vi "R567X_CAN高级功能.vi"() -> ()   [LabVIEW 2020]
panel:
  out "B'":i16
  out "B":i16
  out "A":i16
  out "A'":i16
  out "OK":bool caption="启动标定成功"
  out "完成":bool caption="启动标定成功"
  out "标定成功":bool caption="启动标定成功"
  out "当前扭矩":dbl
  out "扭矩已标定":bool
  out "当前角度":dbl
  out "角度已标定":bool
  out "Out_Time":bool
  in  "error in":errorcluster
  in  "Function":T1(ring)
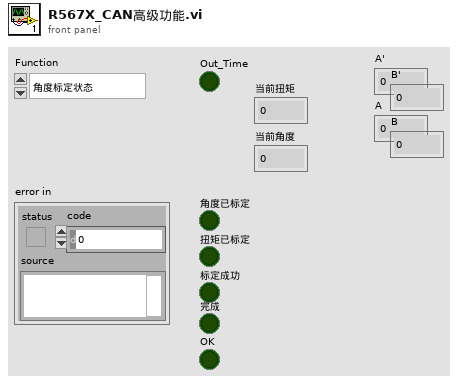
[diagram p1: front panel]
types:
  T1 = enum16{"角度标定状态", "角度标定", "角度标定清除", "扭矩标定状态", "扭矩标定", "扭矩标定清除", "内部软件版本号", "客户软件版本号"}
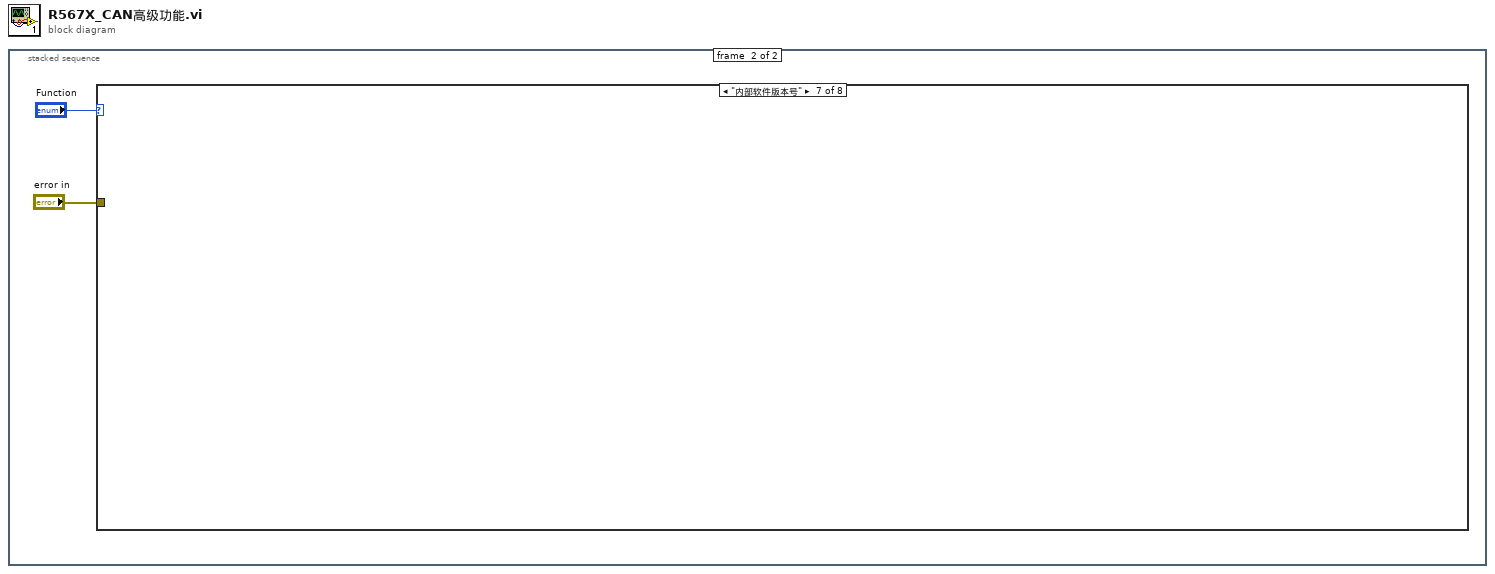
[diagram p0: block diagram]
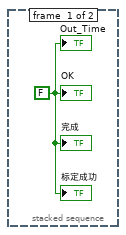
[diagram p2: hidden frame]
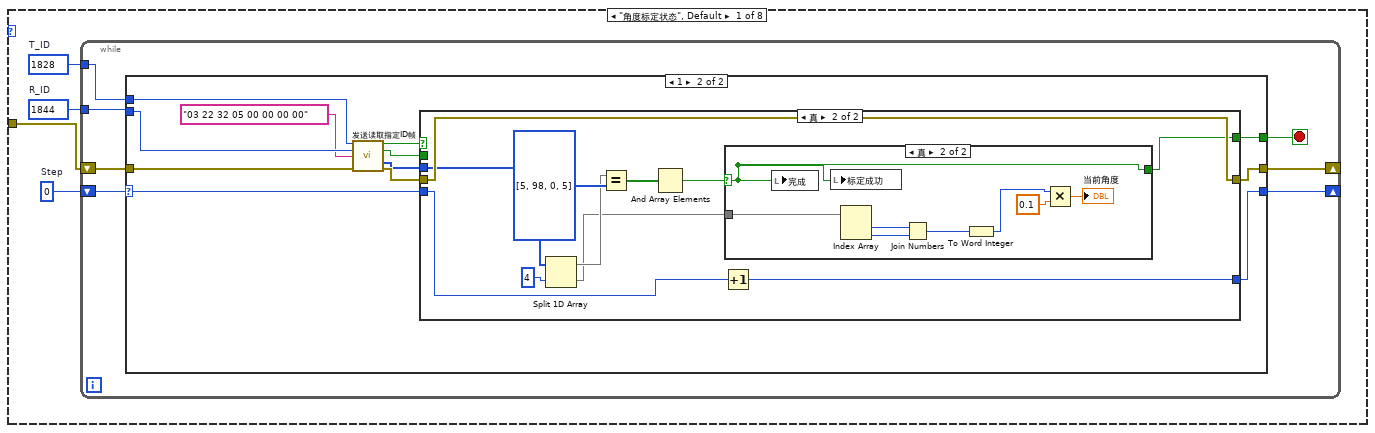
[diagram p3: hidden frame]
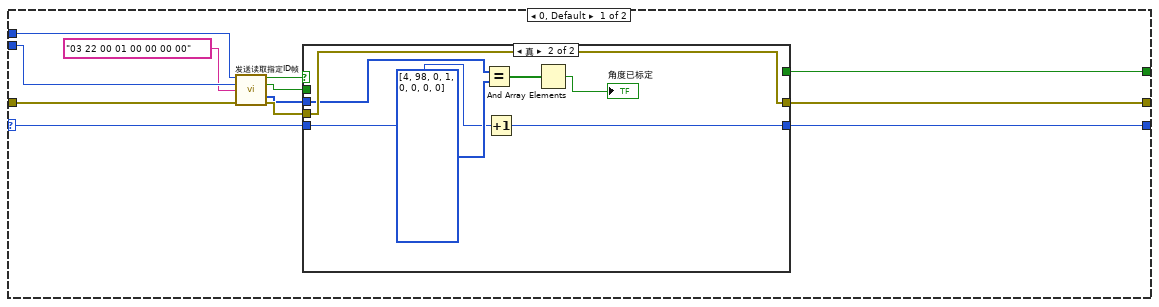
[diagram p4: hidden frame]
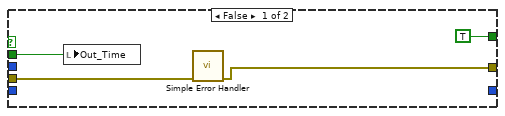
[diagram p5: hidden frame]
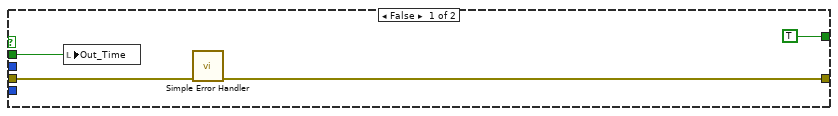
[diagram p6: hidden frame]
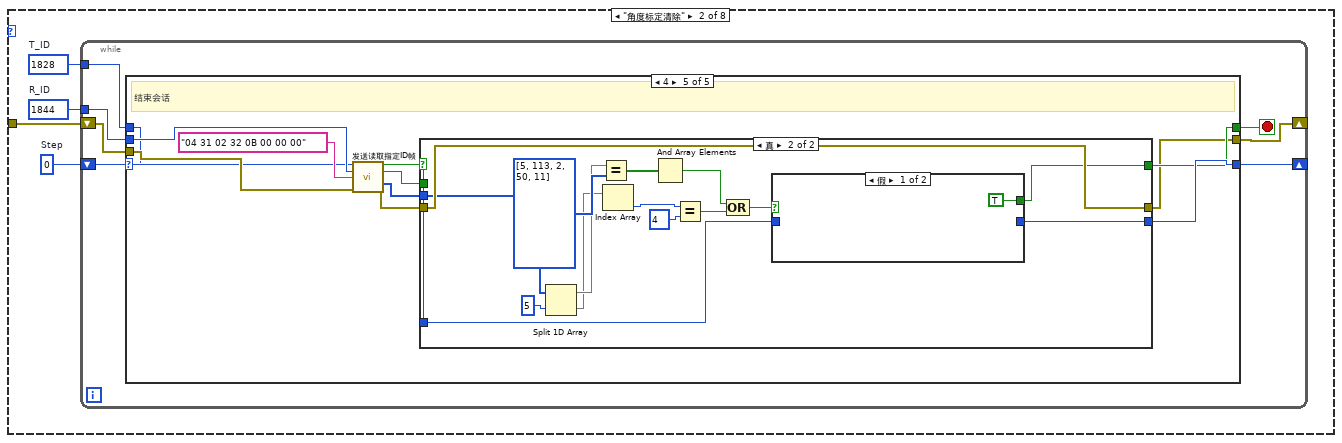
[diagram p8: hidden frame]
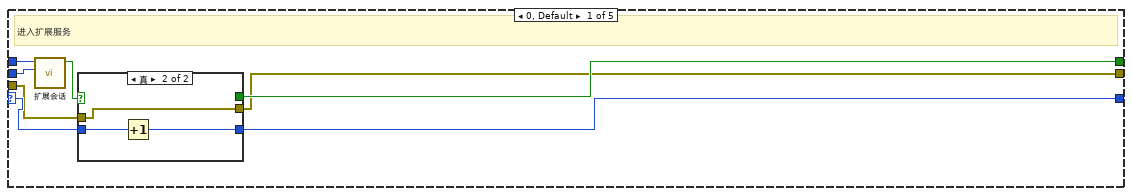
[diagram p9: hidden frame]
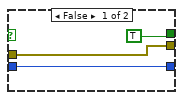
[diagram p10: hidden frame]
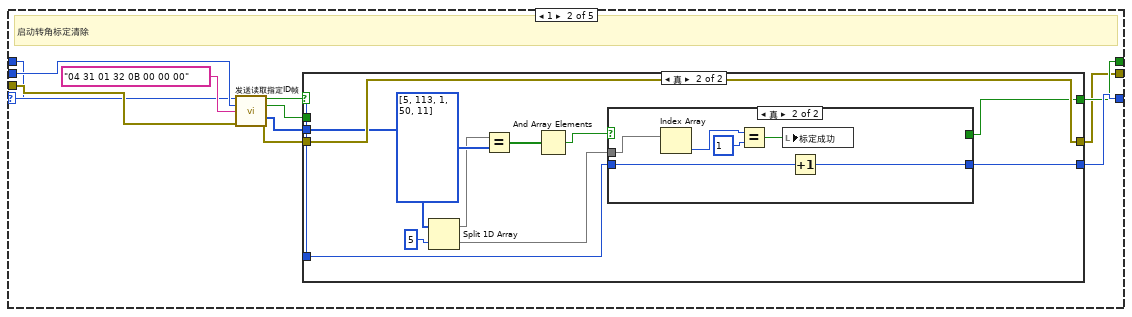
[diagram p11: hidden frame]
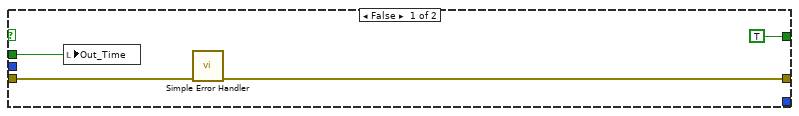
[diagram p12: hidden frame]
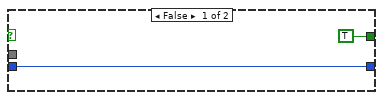
[diagram p13: hidden frame]
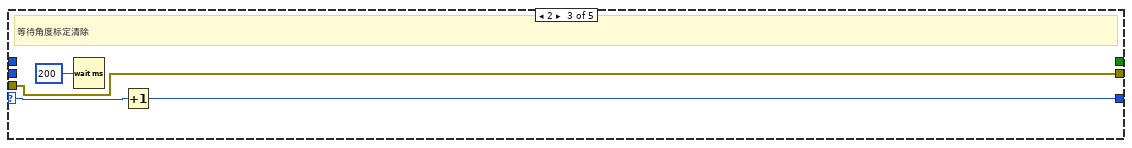
[diagram p14: hidden frame]
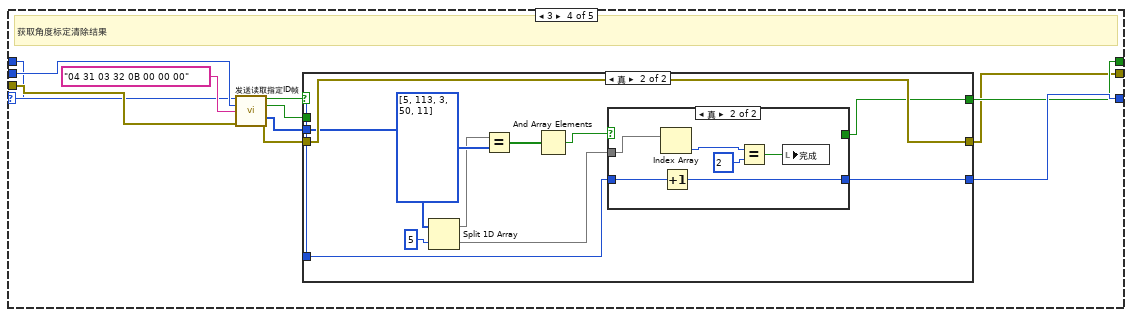
[diagram p15: hidden frame]
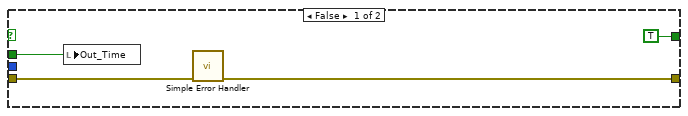
[diagram p16: hidden frame]
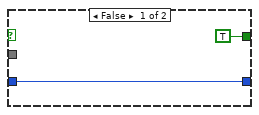
[diagram p17: hidden frame]
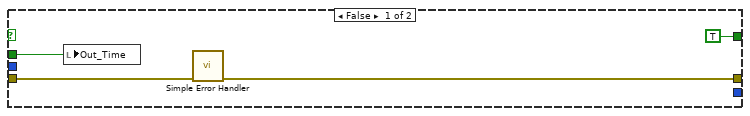
[diagram p18: hidden frame]
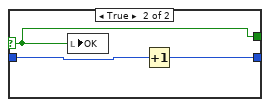
[diagram p19: hidden frame]
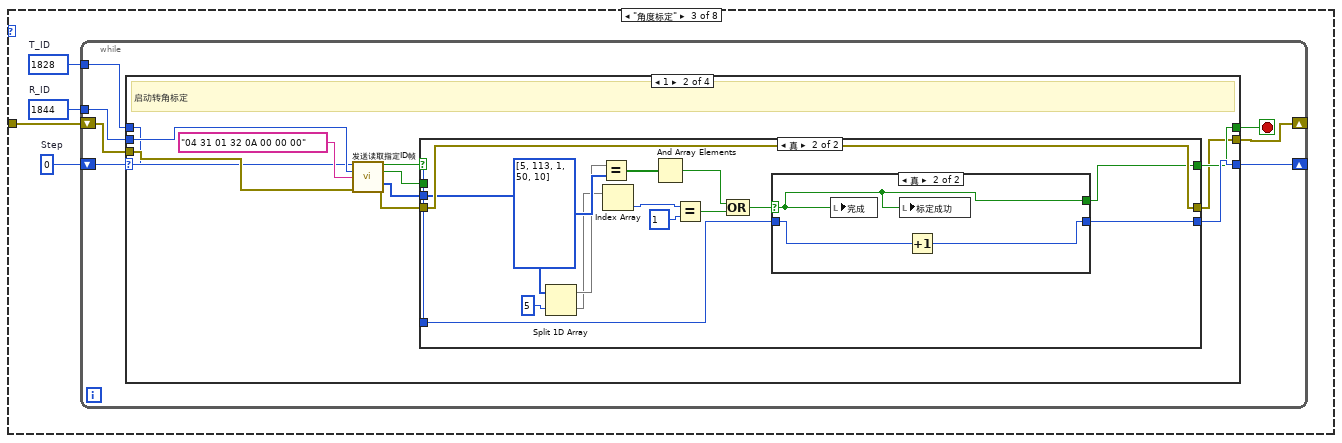
[diagram p20: hidden frame]
diagram:
  n1 = stacked-sequence {
    frame #0 {
      w1 = FALSE ("Out_Time")
      "Out_Time" <- w1
      "标定成功" <- w1
      "完成" <- w1
      "OK" <- w1
    }
    frame #1 {
      n2 = case shown="\"内部软件版本号\"" "Function" {
        tunnel: "error in" -> [w7 w73 w207 w311 w377 w605 _ _]
        frame "角度标定状态", Default {
          w4 = u32 1828  # T_ID
          w5 = u32 1844  # R_ID
          w6 = 0  # Step
          n3 = while {
            tunnel: w4 -> [w14]
            tunnel: w5 -> [w12]
            shift-right: [w8] -> _
            shift-left: w6 -> [w11]
            shift-right: [w9] -> _
            shift-left: w7 -> [w13]
            stop <- w10 stop-if-true
            n4 = case shown="1" w11 {
              selector: w11 -> [w16 w39]
              tunnel: w14 -> [w26 w49]
              tunnel: w13 -> [w25 w48]
              tunnel: w12 -> [w24 w47]
              tunnel: [w20 w43] -> w10
              tunnel: [w18 w41] -> w9
              tunnel: [w15 w38] -> w8
              frame 0, Default {
                n5 = call "发送读取指定ID帧.vi"("T_ID"=w26, "R_ID"=w24, "CAN_Frame"="03 22 00 01 00 00 00 00", "error in (no error)"=w25) -> ("OK"=w22:bool, "Out_Time"=w21:bool, "Recive"=w17:u8[], "error out"=w19:errorcluster)  [unwired: 7 in, 1 out]
                n6 = case shown="真" w22 {
                  tunnel: w21 -> [w30 _]
                  tunnel: [TRUE _] -> w20
                  tunnel: w19 -> [w28 w37]
                  tunnel: [w27 w37] -> w18
                  tunnel: w17 -> [_ w36]
                  tunnel: w16 -> [_ w32]
                  tunnel: [_ w31] -> w15
                  frame False {
                    n7 = local write "Out_Time"(w30) -> ()
                    n8 = call <vilib>:"Simple Error Handler.vi"("error in (no error)"=w28) -> ("error out"=w27:errorcluster)  [unwired: 4 in, 4 out]
                  }
                  frame True {
                    n9 = Equal?(x=w36, y=u8[] [4, 98, 0, 1, 0, 0, 0, 0]) -> (x = y?=w34:bool[])
                    n10 = Increment(x=w32) -> (x+1=w31:i32)
                    n11 = And Array Elements(Boolean array=w34) -> (logical AND=→"角度已标定":bool)
                  }
                }
              }
              frame 1 {
                n12 = call "发送读取指定ID帧.vi"("T_ID"=w49, "R_ID"=w47, "CAN_Frame"="03 22 32 05 00 00 00 00", "error in (no error)"=w48) -> ("OK"=w45:bool, "Out_Time"=w44:bool, "Recive"=w40:u8[], "error out"=w42:errorcluster)  [unwired: 7 in, 1 out]
                n13 = case shown="真" w45 {
                  tunnel: w44 -> [w53 _]
                  tunnel: [TRUE w54] -> w43
                  tunnel: w42 -> [w51 w64]
                  tunnel: [w50 w64] -> w41
                  tunnel: w40 -> [_ w59]
                  tunnel: w39 -> [_ w61]
                  tunnel: [_ w60] -> w38
                  frame False {
                    n14 = local write "Out_Time"(w53) -> ()
                    n15 = call <vilib>:"Simple Error Handler.vi"("error in (no error)"=w51) -> ("error out"=w50:errorcluster)  [unwired: 4 in, 4 out]
                  }
                  frame True {
                    n16 = Split 1D Array(array=w59, index=4 ("索引")) -> (first subarray=w57:u8[], second subarray=w56:u8[])
                    n17 = Equal?(x=w57, y=u8[] [5, 98, 0, 5]) -> (x = y?=w62:bool[])
                    n18 = And Array Elements(Boolean array=w62) -> (logical AND=w55:bool)
                    n19 = Increment(x=w61) -> (x+1=w60:i32)
                    n20 = case shown="真" w55 {
                      selector: w55 -> [_ w65]
                      tunnel: w56 -> [_ w72]
                      tunnel: [_ w65] -> w54
                      frame False {
                      }
                      frame True {
                        n21 = local write "完成"(w65) -> ()
                        n22 = local write "标定成功"(w65) -> ()
                        n23 = Index Array(array=w72) -> (element #1=w70:u8, element #2=w71:u8)  [unwired: 2 in]
                        n24 = Join Numbers(hi=w70, lo=w71) -> ((hi.lo)=w67:u16)
                        n25 = To Word Integer(number=w67) -> (16bit integer=w66:i16)
                        n26 = Multiply(x=w66, y=0.1) -> (x*y=→"当前角度":dbl)
                      }
                    }
                  }
                }
              }
            }
          }
        }
        frame "角度标定清除" {
          w76 = u32 1828  # T_ID
          w75 = u32 1844  # R_ID
          w74 = 0  # Step
          n27 = while {
            tunnel: w76 -> [w83]
            tunnel: w75 -> [w81]
            shift-right: [w77] -> _
            shift-left: w74 -> [w80]
            shift-right: [w78] -> _
            shift-left: w73 -> [w82]
            stop <- w79 stop-if-true
            n28 = case shown="4" w80 {
              selector: w80 -> [w88 w102 w135 w141 w176]
              tunnel: w83 -> [w91 w101 _ w140 w175]
              tunnel: w82 -> [w85 w103 w133 w142 w177]
              tunnel: w81 -> [w90 w104 _ w143 w178]
              tunnel: [w86 w99 _ w138 w173] -> w79
              tunnel: [w84 w98 w133 w137 w172] -> w78
              tunnel: [w87 w100 w134 w139 w174] -> w77
              frame 0, Default {
                # "进入扩展服务"
                n29 = call "扩展会话.vi"("R_ID"=w90, "T_ID"=w91) -> ("OK"=w89:bool)  [unwired: 8 in, 1 out]
                n30 = case shown="真" w89 {
                  tunnel: w88 -> [w94 w97]
                  tunnel: [w94 w96] -> w87
                  tunnel: [TRUE _] -> w86
                  tunnel: [w92 w95] -> w84
                  tunnel: w85 -> [w92 w95]
                  frame False {
                  }
                  frame True {
                    n31 = Increment(x=w97) -> (x+1=w96:i32)
                  }
                }
              }
              frame 1 {
                # "启动转角标定清除"
                n32 = call "发送读取指定ID帧.vi"("T_ID"=w101, "R_ID"=w104, "CAN_Frame"="04 31 01 32 0B 00 00 00", "error in (no error)"=w103) -> ("OK"=w109:bool, "Out_Time"=w108:bool, "Recive"=w106:u8[], "error out"=w107:errorcluster)  [unwired: 7 in, 1 out]
                n33 = case shown="真" w109 {
                  tunnel: w108 -> [w113 _]
                  tunnel: [TRUE w114] -> w99
                  tunnel: w107 -> [w111 w124]
                  tunnel: [w110 w124] -> w98
                  tunnel: w106 -> [_ w121]
                  tunnel: w102 -> [_ w116]
                  tunnel: [_ w115] -> w100
                  frame False {
                    n34 = local write "Out_Time"(w113) -> ()
                    n35 = call <vilib>:"Simple Error Handler.vi"("error in (no error)"=w111) -> ("error out"=w110:errorcluster)  [unwired: 4 in, 4 out]
                  }
                  frame True {
                    n36 = Split 1D Array(array=w121, index=5 ("索引")) -> (first subarray=w119:u8[], second subarray=w118:u8[])
                    n37 = Equal?(x=w119, y=u8[] [5, 113, 1, 50, 11]) -> (x = y?=w122:bool[])
                    n38 = And Array Elements(Boolean array=w122) -> (logical AND=w117:bool)
                    n39 = case shown="真" w117 {
                      tunnel: w118 -> [_ w132]
                      tunnel: w116 -> [w126 w129]
                      tunnel: [w126 w128] -> w115
                      tunnel: [TRUE _] -> w114
                      frame False {
                      }
                      frame True {
                        n40 = Index Array(array=w132) -> (element=w131:u8)  [unwired: 1 in]
                        n41 = Equal?(x=w131, y=u8 1) -> (x = y?=w127:bool)
                        n42 = local write "标定成功"(w127) -> ()
                        n43 = Increment(x=w129) -> (x+1=w128:i32)
                      }
                    }
                  }
                }
              }
              frame 2 {
                # "等待角度标定清除"
                n44 = Wait (ms)(milliseconds to wait=u32 200 ("等待时间（毫秒）")) -> ()  [unwired: 1 out]
                n45 = Increment(x=w135) -> (x+1=w134:i32)
              }
              frame 3 {
                # "获取角度标定清除结果"
                n46 = call "发送读取指定ID帧.vi"("T_ID"=w140, "R_ID"=w143, "CAN_Frame"="04 31 03 32 0B 00 00 00", "error in (no error)"=w142) -> ("OK"=w148:bool, "Out_Time"=w147:bool, "Recive"=w145:u8[], "error out"=w146:errorcluster)  [unwired: 7 in, 1 out]
                n47 = case shown="真" w148 {
                  tunnel: w147 -> [w152 _]
                  tunnel: [TRUE w153] -> w138
                  tunnel: w146 -> [w150 w163]
                  tunnel: [w149 w163] -> w137
                  tunnel: w145 -> [_ w160]
                  tunnel: w141 -> [_ w155]
                  tunnel: [_ w154] -> w139
                  frame False {
                    n48 = local write "Out_Time"(w152) -> ()
                    n49 = call <vilib>:"Simple Error Handler.vi"("error in (no error)"=w150) -> ("error out"=w149:errorcluster)  [unwired: 4 in, 4 out]
                  }
                  frame True {
                    n50 = Split 1D Array(array=w160, index=5 ("索引")) -> (first subarray=w158:u8[], second subarray=w157:u8[])
                    n51 = Equal?(x=w158, y=u8[] [5, 113, 3, 50, 11]) -> (x = y?=w161:bool[])
                    n52 = And Array Elements(Boolean array=w161) -> (logical AND=w156:bool)
                    n53 = case shown="真" w156 {
                      tunnel: w157 -> [_ w171]
                      tunnel: w155 -> [w165 w168]
                      tunnel: [w165 w167] -> w154
                      tunnel: [TRUE _] -> w153
                      frame False {
                      }
                      frame True {
                        n54 = Index Array(array=w171) -> (element=w170:u8)  [unwired: 1 in]
                        n55 = Increment(x=w168) -> (x+1=w167:i32)
                        n56 = Equal?(x=w170, y=u8 2) -> (x = y?=w166:bool)
                        n57 = local write "完成"(w166) -> ()
                      }
                    }
                  }
                }
              }
              frame 4 {
                # "结束会话"
                n58 = call "发送读取指定ID帧.vi"("T_ID"=w175, "R_ID"=w178, "CAN_Frame"="04 31 02 32 0B 00 00 00", "error in (no error)"=w177) -> ("OK"=w183:bool, "Out_Time"=w182:bool, "Recive"=w180:u8[], "error out"=w181:errorcluster)  [unwired: 7 in, 1 out]
                n59 = case shown="真" w183 {
                  tunnel: w182 -> [w187 _]
                  tunnel: [TRUE w195] -> w173
                  tunnel: w181 -> [w185 w202]
                  tunnel: [w184 w202] -> w172
                  tunnel: w180 -> [_ w199]
                  tunnel: w176 -> [_ w191]
                  tunnel: [_ w190] -> w174
                  frame False {
                    n60 = local write "Out_Time"(w187) -> ()
                    n61 = call <vilib>:"Simple Error Handler.vi"("error in (no error)"=w185) -> ("error out"=w184:errorcluster)  [unwired: 4 in, 4 out]
                  }
                  frame True {
                    n62 = Split 1D Array(array=w199, index=5 ("索引")) -> (first subarray=w197:u8[], second subarray=w192:u8[])
                    n63 = Equal?(x=w197, y=u8[] [5, 113, 2, 50, 11]) -> (x = y?=w200:bool[])
                    n64 = Index Array(array=w192) -> (element=w194:u8)  [unwired: 1 in]
                    n65 = And Array Elements(Boolean array=w200) -> (logical AND=w196:bool)
                    n66 = Equal?(x=w194, y=u8 4) -> (x = y?=w188:bool)
                    n67 = Compound Arithmetic op=OR ("复合运算")(w196, w188) -> (w189:bool)
                    n68 = case shown="假" w189 {
                      selector: w189 -> [_ w206]
                      tunnel: [TRUE w206] -> w195
                      tunnel: w191 -> [_ w205]
                      tunnel: [_ w204] -> w190
                      frame False {
                      }
                      frame True {
                        n69 = local write "OK"(w206) -> ()
                        n70 = Increment(x=w205) -> (x+1=w204:i32)
                      }
                    }
                  }
                }
              }
            }
          }
        }
        frame "角度标定" {
          w210 = u32 1828  # T_ID
          w209 = u32 1844  # R_ID
          w208 = 0  # Step
          n71 = while {
            tunnel: w210 -> [w217]
            tunnel: w209 -> [w215]
            shift-right: [w211] -> _
            shift-left: w208 -> [w214]
            shift-right: [w212] -> _
            shift-left: w207 -> [w216]
            stop <- w213 stop-if-true
            n72 = case shown="1" w214 {
              selector: w214 -> [w222 w236 w270 w276]
              tunnel: w217 -> [w225 w235 _ w275]
              tunnel: w216 -> [w219 w237 w268 w277]
              tunnel: w215 -> [w224 w238 _ w278]
              tunnel: [w220 w233 _ w273] -> w213
              tunnel: [w218 w232 w268 w272] -> w212
              tunnel: [w221 w234 w269 w274] -> w211
              frame 0, Default {
                # "进入扩展服务"
                n73 = call "扩展会话.vi"("R_ID"=w224, "T_ID"=w225) -> ("OK"=w223:bool)  [unwired: 8 in, 1 out]
                n74 = case shown="真" w223 {
                  tunnel: w222 -> [w228 w231]
                  tunnel: [w228 w230] -> w221
                  tunnel: [TRUE _] -> w220
                  tunnel: [w226 w229] -> w218
                  tunnel: w219 -> [w226 w229]
                  frame False {
                  }
                  frame True {
                    n75 = Increment(x=w231) -> (x+1=w230:i32)
                  }
                }
              }
              frame 1 {
                # "启动转角标定"
                n76 = call "发送读取指定ID帧.vi"("T_ID"=w235, "R_ID"=w238, "CAN_Frame"="04 31 01 32 0A 00 00 00", "error in (no error)"=w237) -> ("OK"=w243:bool, "Out_Time"=w242:bool, "Recive"=w240:u8[], "error out"=w241:errorcluster)  [unwired: 7 in, 1 out]
                n77 = case shown="真" w243 {
                  tunnel: w242 -> [w247 _]
                  tunnel: [TRUE w253] -> w233
                  tunnel: w241 -> [w245 w262]
                  tunnel: [w244 w262] -> w232
                  tunnel: w240 -> [_ w259]
                  tunnel: w236 -> [_ w255]
                  tunnel: [_ w254] -> w234
                  frame False {
                    n78 = local write "Out_Time"(w247) -> ()
                    n79 = call <vilib>:"Simple Error Handler.vi"("error in (no error)"=w245) -> ("error out"=w244:errorcluster)  [unwired: 4 in, 4 out]
                  }
                  frame True {
                    n80 = Split 1D Array(array=w259, index=5 ("索引")) -> (first subarray=w257:u8[], second subarray=w250:u8[])
                    n81 = Equal?(x=w257, y=u8[] [5, 113, 1, 50, 10]) -> (x = y?=w260:bool[])
                    n82 = Index Array(array=w250) -> (element=w252:u8)  [unwired: 1 in]
                    n83 = And Array Elements(Boolean array=w260) -> (logical AND=w256:bool)
                    n84 = Equal?(x=w252, y=u8 1) -> (x = y?=w248:bool)
                    n85 = Compound Arithmetic op=OR ("复合运算")(w256, w248) -> (w249:bool)
                    n86 = case shown="真" w249 {
                      selector: w249 -> [_ w265]
                      tunnel: w255 -> [w264 w267]
                      tunnel: [w264 w266] -> w254
                      tunnel: [TRUE w265] -> w253
                      frame False {
                      }
                      frame True {
                        n87 = local write "完成"(w265) -> ()
                        n88 = local write "标定成功"(w265) -> ()
                        n89 = Increment(x=w267) -> (x+1=w266:i32)
                      }
                    }
                  }
                }
              }
              frame 2 {
                # "等待角度标定"
                n90 = Wait (ms)(milliseconds to wait=u32 200 ("等待时间（毫秒）")) -> ()  [unwired: 1 out]
                n91 = Increment(x=w270) -> (x+1=w269:i32)
              }
              frame 3 {
                # "获取角度标定结果"
                n92 = call "发送读取指定ID帧.vi"("T_ID"=w275, "R_ID"=w278, "CAN_Frame"="04 31 02 32 0A 00 00 00", "error in (no error)"=w277) -> ("OK"=w283:bool, "Out_Time"=w282:bool, "Recive"=w280:u8[], "error out"=w281:errorcluster)  [unwired: 7 in, 1 out]
                n93 = case shown="真" w283 {
                  tunnel: w282 -> [w287 _]
                  tunnel: [TRUE w288] -> w273
                  tunnel: w281 -> [w285 w298]
                  tunnel: [w284 w298] -> w272
                  tunnel: w280 -> [_ w295]
                  tunnel: w276 -> [_ w290]
                  tunnel: [_ w289] -> w274
                  frame False {
                    n94 = local write "Out_Time"(w287) -> ()
                    n95 = call <vilib>:"Simple Error Handler.vi"("error in (no error)"=w285) -> ("error out"=w284:errorcluster)  [unwired: 4 in, 4 out]
                  }
                  frame True {
                    n96 = Split 1D Array(array=w295, index=5 ("索引")) -> (first subarray=w293:u8[], second subarray=w292:u8[])
                    n97 = Equal?(x=w293, y=u8[] [5, 113, 2, 50, 10]) -> (x = y?=w296:bool[])
                    n98 = And Array Elements(Boolean array=w296) -> (logical AND=w291:bool)
                    n99 = case shown="真" w291 {
                      tunnel: w292 -> [_ w307]
                      tunnel: w290 -> [w300 w304]
                      tunnel: [w300 w303] -> w289
                      tunnel: [TRUE TRUE] -> w288
                      frame False {
                      }
                      frame True {
                        n100 = Index Array(array=w307) -> (element=w306:u8)  [unwired: 1 in]
                        n101 = Increment(x=w304) -> (x+1=w303:i32)
                        n102 = Equal?(x=w306, y=u8 4) -> (x = y?=w302:bool)
                        n103 = local write "完成"(w302) -> ()
                      }
                    }
                  }
                }
              }
            }
          }
        }
        frame "扭矩标定状态" {
          w308 = u32 1828  # T_ID
          w309 = u32 1844  # R_ID
          w310 = 0  # Step
          n104 = while {
            tunnel: w308 -> [w318]
            tunnel: w309 -> [w316]
            shift-right: [w312] -> _
            shift-left: w310 -> [w315]
            shift-right: [w313] -> _
            shift-left: w311 -> [w317]
            stop <- w314 stop-if-true
            n105 = case shown="1" w315 {
              selector: w315 -> [w320 w343]
              tunnel: w318 -> [w330 w353]
              tunnel: w317 -> [w329 w352]
              tunnel: w316 -> [w328 w351]
              tunnel: [w324 w347] -> w314
              tunnel: [w322 w345] -> w313
              tunnel: [w319 w342] -> w312
              frame 0, Default {
                n106 = call "发送读取指定ID帧.vi"("T_ID"=w330, "R_ID"=w328, "CAN_Frame"="03 22 00 05 00 00 00 00", "error in (no error)"=w329) -> ("OK"=w326:bool, "Out_Time"=w325:bool, "Recive"=w321:u8[], "error out"=w323:errorcluster)  [unwired: 7 in, 1 out]
                n107 = case shown="真" w326 {
                  tunnel: w325 -> [w334 _]
                  tunnel: [TRUE _] -> w324
                  tunnel: w323 -> [w332 w341]
                  tunnel: [w331 w341] -> w322
                  tunnel: w321 -> [_ w340]
                  tunnel: w320 -> [_ w336]
                  tunnel: [_ w335] -> w319
                  frame False {
                    n108 = local write "Out_Time"(w334) -> ()
                    n109 = call <vilib>:"Simple Error Handler.vi"("error in (no error)"=w332) -> ("error out"=w331:errorcluster)  [unwired: 4 in, 4 out]
                  }
                  frame True {
                    n110 = Equal?(x=w340, y=u8[] [4, 98, 0, 5, 0, 0, 0, 0]) -> (x = y?=w338:bool[])
                    n111 = Increment(x=w336) -> (x+1=w335:i32)
                    n112 = And Array Elements(Boolean array=w338) -> (logical AND=→"扭矩已标定":bool)
                  }
                }
              }
              frame 1 {
                n113 = call "发送读取指定ID帧.vi"("T_ID"=w353, "R_ID"=w351, "CAN_Frame"="03 22 32 02 00 00 00 00", "error in (no error)"=w352) -> ("OK"=w349:bool, "Out_Time"=w348:bool, "Recive"=w344:u8[], "error out"=w346:errorcluster)  [unwired: 7 in, 1 out]
                n114 = case shown="真" w349 {
                  tunnel: w348 -> [w357 _]
                  tunnel: [TRUE w358] -> w347
                  tunnel: w346 -> [w355 w368]
                  tunnel: [w354 w368] -> w345
                  tunnel: w344 -> [_ w363]
                  tunnel: w343 -> [_ w365]
                  tunnel: [_ w364] -> w342
                  frame False {
                    n115 = local write "Out_Time"(w357) -> ()
                    n116 = call <vilib>:"Simple Error Handler.vi"("error in (no error)"=w355) -> ("error out"=w354:errorcluster)  [unwired: 4 in, 4 out]
                  }
                  frame True {
                    n117 = Split 1D Array(array=w363, index=4 ("索引")) -> (first subarray=w361:u8[], second subarray=w360:u8[])
                    n118 = Equal?(x=w361, y=u8[] [5, 98, 0, 2]) -> (x = y?=w366:bool[])
                    n119 = And Array Elements(Boolean array=w366) -> (logical AND=w359:bool)
                    n120 = Increment(x=w365) -> (x+1=w364:i32)
                    n121 = case shown="真" w359 {
                      selector: w359 -> [_ w369]
                      tunnel: w360 -> [_ w376]
                      tunnel: [_ w369] -> w358
                      frame False {
                      }
                      frame True {
                        n122 = local write "完成"(w369) -> ()
                        n123 = Index Array(array=w376) -> (element #1=w374:u8, element #2=w375:u8)  [unwired: 2 in]
                        n124 = Join Numbers(hi=w374, lo=w375) -> ((hi.lo)=w371:u16)
                        n125 = To Word Integer(number=w371) -> (16bit integer=w370:i16)
                        n126 = Multiply(x=w370, y=0.0009765625) -> (x*y=→"当前扭矩":dbl)
                      }
                    }
                  }
                }
              }
            }
          }
        }
        frame "扭矩标定" {
          w378 = u32 1828  # T_ID
          w379 = u32 1844  # R_ID
          w380 = 0  # Step
          n127 = while {
            tunnel: w378 -> [w387]
            tunnel: w379 -> [w385]
            shift-right: [w381] -> _
            shift-left: w380 -> [w384]
            shift-right: [w382] -> _
            shift-left: w377 -> [w386]
            stop <- w383 stop-if-true
            n128 = case shown="6" w384 {
              selector: w384 -> [w389 w427 _ w476 w509 w541 w577]
              tunnel: w387 -> [w399 w437 w470 w492 w525 w551 w587]
              tunnel: w386 -> [w398 w436 w468 w482 w515 w550 w586]
              tunnel: w385 -> [w397 w435 w469 w491 w524 w549 w585]
              tunnel: [w393 w431 w464 w474 w507 w545 w581] -> w383
              tunnel: [w391 w429 w465 w478 w511 w543 w579] -> w382
              tunnel: [w388 w426 _ w475 w508 w540 w576] -> w381
              frame 0, Default {
                # "读取T1原始值A"
                n129 = call "发送读取指定ID帧.vi"("T_ID"=w399, "R_ID"=w397, "CAN_Frame"="03 22 07 00 00 00 00 00", "error in (no error)"=w398) -> ("OK"=w395:bool, "Out_Time"=w394:bool, "Recive"=w390:u8[], "error out"=w392:errorcluster)  [unwired: 7 in, 1 out]
                n130 = case shown="真" w395 {
                  tunnel: w394 -> [w403 _]
                  tunnel: [TRUE w404] -> w393
                  tunnel: w392 -> [w401 w414]
                  tunnel: [w400 w414] -> w391
                  tunnel: w390 -> [_ w411]
                  tunnel: w389 -> [_ w406]
                  tunnel: [_ w405] -> w388
                  frame False {
                    n131 = local write "Out_Time"(w403) -> ()
                    n132 = call <vilib>:"Simple Error Handler.vi"("error in (no error)"=w401) -> ("error out"=w400:errorcluster)  [unwired: 4 in, 4 out]
                  }
                  frame True {
                    n133 = Split 1D Array(array=w411, index=4 ("索引")) -> (first subarray=w409:u8[], second subarray=w408:u8[])
                    n134 = Equal?(x=w409, y=u8[] [5, 98, 7, 0]) -> (x = y?=w412:bool[])
                    n135 = And Array Elements(Boolean array=w412) -> (logical AND=w407:bool)
                    n136 = case shown="假" w407 {
                      tunnel: w408 -> [_ w425]
                      tunnel: w406 -> [w415 w418]
                      tunnel: [w415 w417] -> w405
                      tunnel: [TRUE _] -> w404
                      frame False {
                      }
                      frame True {
                        n137 = Index Array(array=w425) -> (element #1=w423:u8, element #2=w424:u8)  [unwired: 2 in]
                        n138 = Join Numbers(hi=w423, lo=w424) -> ((hi.lo)=w422:u16)
                        n139 = Increment(x=w418) -> (x+1=w417:i32)
                        n140 = To Word Integer(number=w422) -> (16bit integer=w421:i16)
                        "A" <- w421
                        n141 = Subtract(x=i16 16384 ("16位整型"), y=w421) -> (x-y=→"A'":i16)
                      }
                    }
                  }
                }
              }
              frame 1 {
                # "读取T2原始值B"
                n142 = call "发送读取指定ID帧.vi"("T_ID"=w437, "R_ID"=w435, "CAN_Frame"="03 22 07 01 00 00 00 00", "error in (no error)"=w436) -> ("OK"=w433:bool, "Out_Time"=w432:bool, "Recive"=w428:u8[], "error out"=w430:errorcluster)  [unwired: 7 in, 1 out]
                n143 = case shown="真" w433 {
                  tunnel: w432 -> [w441 _]
                  tunnel: [TRUE w442] -> w431
                  tunnel: w430 -> [w439 w452]
                  tunnel: [w438 w452] -> w429
                  tunnel: w428 -> [_ w449]
                  tunnel: w427 -> [_ w444]
                  tunnel: [_ w443] -> w426
                  frame False {
                    n144 = local write "Out_Time"(w441) -> ()
                    n145 = call <vilib>:"Simple Error Handler.vi"("error in (no error)"=w439) -> ("error out"=w438:errorcluster)  [unwired: 4 in, 4 out]
                  }
                  frame True {
                    n146 = Split 1D Array(array=w449, index=4 ("索引")) -> (first subarray=w447:u8[], second subarray=w446:u8[])
                    n147 = Equal?(x=w447, y=u8[] [5, 98, 7, 1]) -> (x = y?=w450:bool[])
                    n148 = And Array Elements(Boolean array=w450) -> (logical AND=w445:bool)
                    n149 = case shown="真" w445 {
                      tunnel: w446 -> [_ w463]
                      tunnel: w444 -> [w453 w456]
                      tunnel: [w453 w455] -> w443
                      tunnel: [TRUE _] -> w442
                      frame False {
                      }
                      frame True {
                        n150 = Increment(x=w456) -> (x+1=w455:i32)
                        n151 = Index Array(array=w463) -> (element #1=w461:u8, element #2=w462:u8)  [unwired: 2 in]
                        n152 = Join Numbers(hi=w461, lo=w462) -> ((hi.lo)=w460:u16)
                        n153 = To Word Integer(number=w460) -> (16bit integer=w459:i16)
                        "B" <- w459
                        n154 = Subtract(x=i16 16384 ("16位整型"), y=w459) -> (x-y=→"B'":i16)
                      }
                    }
                  }
                }
              }
              frame 2 {
                # "进入扩展会话"
                n155 = call "扩展会话.vi"("error in"=w468, "R_ID"=w469, "T_ID"=w470) -> ("error out"=w466:errorcluster, "OK"=w467:bool)  [unwired: 7 in]
                n156 = case shown="真" w467 {
                  tunnel: w466 -> [w472 w473]
                  tunnel: [w472 w473] -> w465
                  tunnel: [TRUE _] -> w464
                  frame False {
                  }
                  frame True {
                  }
                }
              }
              frame 3 {
                w486 = i16 2 ("宽度(-)")
                # "写入T1标定值A'"
                n157 = local read "A'"() -> (w489:i16)
                n158 = Split Number(x=w489) -> (hi(x)=w488:u8, lo(x)=w487:u8)
                n159 = Number To Hexadecimal String(1:w486, 2:w488) -> (0:w485:string)
                n160 = Number To Hexadecimal String(1:w486, 2:w487) -> (0:w484:string)
                n161 = Format Into String(format string="10 09 31 1 33 01 %s %s" ("格式字符串"), w485, w484) -> (resulting string=w483:string)  [unwired: 2 in, 1 out]
                n162 = call "发送读取指定ID帧.vi"("T_ID"=w492, "R_ID"=w491, "CAN_Frame"=w483, "error in (no error)"=w482) -> ("OK"=w481:bool, "Out_Time"=w480:bool, "Recive"=w477:u8[], "error out"=w479:errorcluster)  [unwired: 7 in, 1 out]
                n163 = case shown="真" w481 {
                  tunnel: w480 -> [w495 _]
                  tunnel: w479 -> [w494 w497]
                  tunnel: [w493 w497] -> w478
                  tunnel: w477 -> [_ w501]
                  tunnel: w476 -> [_ w499]
                  tunnel: [_ w498] -> w475
                  tunnel: [_ w496] -> w474
                  frame False {
                    n164 = local write "Out_Time"(w495) -> ()
                    n165 = call <vilib>:"Simple Error Handler.vi"("error in (no error)"=w494) -> ("error out"=w493:errorcluster)  [unwired: 4 in, 4 out]
                  }
                  frame True {
                    n166 = Equal?(x=w501, y=u8[] [48, 0, 10, 0, 0, 0, 0, 0]) -> (x = y?=w503:bool[])
                    n167 = And Array Elements(Boolean array=w503) -> (logical AND=w500:bool)
                    n168 = case shown="假" w500 {
                      tunnel: w499 -> [_ w506]
                      tunnel: [_ w505] -> w498
                      tunnel: [TRUE _] -> w496
                      frame False {
                      }
                      frame True {
                        n169 = Increment(x=w506) -> (x+1=w505:i32)
                      }
                    }
                  }
                }
              }
              frame 4 {
                w519 = i16 2 ("宽度(-)")
                # "写入T2标定值B'"
                n170 = local read "B'"() -> (w522:i16)
                n171 = Split Number(x=w522) -> (hi(x)=w521:u8, lo(x)=w520:u8)
                n172 = Number To Hexadecimal String(1:w519, 2:w521) -> (0:w518:string)
                n173 = Number To Hexadecimal String(1:w519, 2:w520) -> (0:w517:string)
                n174 = Format Into String(format string="21 %s %s 00 00 00 00 00" ("格式字符串"), w518, w517) -> (resulting string=w516:string)  [unwired: 2 in, 1 out]
                n175 = call "发送读取指定ID帧.vi"("T_ID"=w525, "R_ID"=w524, "CAN_Frame"=w516, "error in (no error)"=w515) -> ("OK"=w514:bool, "Out_Time"=w513:bool, "Recive"=w510:u8[], "error out"=w512:errorcluster)  [unwired: 7 in, 1 out]
                n176 = case shown="真" w514 {
                  tunnel: w513 -> [w528 _]
                  tunnel: w512 -> [w527 w530]
                  tunnel: [w526 w530] -> w511
                  tunnel: w510 -> [_ w534]
                  tunnel: w509 -> [_ w532]
                  tunnel: [_ w531] -> w508
                  tunnel: [_ w529] -> w507
                  frame False {
                    n177 = local write "Out_Time"(w528) -> ()
                    n178 = call <vilib>:"Simple Error Handler.vi"("error in (no error)"=w527) -> ("error out"=w526:errorcluster)  [unwired: 4 in, 4 out]
                  }
                  frame True {
                    n179 = Equal?(x=w534, y=u8[] [5, 113, 1, 51, 1, 1, 0, 0]) -> (x = y?=w536:bool[])
                    n180 = And Array Elements(Boolean array=w536) -> (logical AND=w533:bool)
                    n181 = case shown="假" w533 {
                      tunnel: w532 -> [_ w539]
                      tunnel: [_ w538] -> w531
                      tunnel: [TRUE _] -> w529
                      frame False {
                      }
                      frame True {
                        n182 = Increment(x=w539) -> (x+1=w538:i32)
                      }
                    }
                  }
                }
              }
              frame 5 {
                # "读取标定状态"
                n183 = call "发送读取指定ID帧.vi"("T_ID"=w551, "R_ID"=w549, "CAN_Frame"="04 31 03 33 01 00 00 00", "error in (no error)"=w550) -> ("OK"=w547:bool, "Out_Time"=w546:bool, "Recive"=w542:u8[], "error out"=w544:errorcluster)  [unwired: 7 in, 1 out]
                n184 = case shown="真" w547 {
                  tunnel: w546 -> [w555 _]
                  tunnel: [TRUE w561] -> w545
                  tunnel: w544 -> [w553 w570]
                  tunnel: [w552 w570] -> w543
                  tunnel: w542 -> [_ w567]
                  tunnel: w541 -> [_ w563]
                  tunnel: [_ w562] -> w540
                  frame False {
                    n185 = local write "Out_Time"(w555) -> ()
                    n186 = call <vilib>:"Simple Error Handler.vi"("error in (no error)"=w553) -> ("error out"=w552:errorcluster)  [unwired: 4 in, 4 out]
                  }
                  frame True {
                    n187 = Split 1D Array(array=w567, index=5 ("索引")) -> (first subarray=w565:u8[], second subarray=w558:u8[])
                    n188 = Equal?(x=w565, y=u8[] [5, 113, 3, 51, 1]) -> (x = y?=w568:bool[])
                    n189 = Index Array(array=w558) -> (element=w560:u8)  [unwired: 1 in]
                    n190 = And Array Elements(Boolean array=w568) -> (logical AND=w564:bool)
                    n191 = Equal?(x=w560, y=u8 1 ("数值")) -> (x = y?=w556:bool)
                    n192 = Compound Arithmetic op=OR ("复合运算")(w564, w556) -> (w557:bool)
                    n193 = case shown="真" w557 {
                      selector: w557 -> [_ w573]
                      tunnel: w563 -> [w571 w575]
                      tunnel: [w571 w574] -> w562
                      tunnel: [TRUE _] -> w561
                      frame False {
                      }
                      frame True {
                        n194 = local write "标定成功"(w573) -> ()
                        n195 = Increment(x=w575) -> (x+1=w574:i32)
                      }
                    }
                  }
                }
              }
              frame 6 {
                # "复位MCU"
                n196 = call "发送读取指定ID帧.vi"("T_ID"=w587, "R_ID"=w585, "CAN_Frame"="02 11 01 00 00 00 00 00", "error in (no error)"=w586) -> ("OK"=w583:bool, "Out_Time"=w582:bool, "Recive"=w578:u8[], "error out"=w580:errorcluster)  [unwired: 7 in, 1 out]
                n197 = case shown="真" w583 {
                  tunnel: w582 -> [w591 _]
                  tunnel: [TRUE w593] -> w581
                  tunnel: w580 -> [w589 w599]
                  tunnel: [w588 w599] -> w579
                  tunnel: w578 -> [_ w596]
                  tunnel: w577 -> [_ w595]
                  tunnel: [_ w594] -> w576
                  frame False {
                    n198 = local write "Out_Time"(w591) -> ()
                    n199 = call <vilib>:"Simple Error Handler.vi"("error in (no error)"=w589) -> ("error out"=w588:errorcluster)  [unwired: 4 in, 4 out]
                  }
                  frame True {
                    n200 = Equal?(x=w596, y=u8[] [2, 81, 1, 0, 0, 0, 0, 0]) -> (x = y?=w597:bool[])
                    n201 = And Array Elements(Boolean array=w597) -> (logical AND=w592:bool)
                    n202 = case shown="真" w592 {
                      selector: w592 -> [_ w602]
                      tunnel: w595 -> [w600 w604]
                      tunnel: [w600 w603] -> w594
                      tunnel: [TRUE w602] -> w593
                      frame False {
                      }
                      frame True {
                        n203 = local write "完成"(w602) -> ()
                        n204 = Increment(x=w604) -> (x+1=w603:i32)
                      }
                    }
                  }
                }
              }
            }
          }
        }
        frame "扭矩标定清除" {
          w608 = u32 1828  # T_ID
          w607 = u32 1844  # R_ID
          w606 = 0  # Step
          n205 = while {
            tunnel: w608 -> [w615]
            tunnel: w607 -> [w613]
            shift-right: [w609] -> _
            shift-left: w606 -> [w612]
            shift-right: [w610] -> _
            shift-left: w605 -> [w614]
            stop <- w611 stop-if-true
            n206 = case shown="1" w612 {
              selector: w612 -> [w620 w634]
              tunnel: w615 -> [w623 w633]
              tunnel: w614 -> [w617 w635]
              tunnel: w613 -> [w622 w636]
              tunnel: [w618 w631] -> w611
              tunnel: [w616 w630] -> w610
              tunnel: [w619 w632] -> w609
              frame 0, Default {
                # "进入扩展服务"
                n207 = call "扩展会话.vi"("R_ID"=w622, "T_ID"=w623) -> ("OK"=w621:bool)  [unwired: 8 in, 1 out]
                n208 = case shown="真" w621 {
                  tunnel: w620 -> [w626 w629]
                  tunnel: [w626 w628] -> w619
                  tunnel: [TRUE _] -> w618
                  tunnel: [w624 w627] -> w616
                  tunnel: w617 -> [w624 w627]
                  frame False {
                  }
                  frame True {
                    n209 = Increment(x=w629) -> (x+1=w628:i32)
                  }
                }
              }
              frame 1 {
                # "启动转角标定清除"
                n210 = call "发送读取指定ID帧.vi"("T_ID"=w633, "R_ID"=w636, "CAN_Frame"="04 2E 07 05 01 00 00 00", "error in (no error)"=w635) -> ("OK"=w641:bool, "Out_Time"=w640:bool, "Recive"=w638:u8[], "error out"=w639:errorcluster)  [unwired: 7 in, 1 out]
                n211 = case shown="真" w641 {
                  tunnel: w640 -> [w645 _]
                  tunnel: [TRUE w646] -> w631
                  tunnel: w639 -> [w643 w653]
                  tunnel: [w642 w653] -> w630
                  tunnel: w638 -> [_ w650]
                  tunnel: w634 -> [_ w648]
                  tunnel: [_ w647] -> w632
                  frame False {
                    n212 = local write "Out_Time"(w645) -> ()
                    n213 = call <vilib>:"Simple Error Handler.vi"("error in (no error)"=w643) -> ("error out"=w642:errorcluster)  [unwired: 4 in, 4 out]
                  }
                  frame True {
                    n214 = Equal?(x=w650, y=u8[] [3, 110, 7, 5, 0, 0, 0, 0]) -> (x = y?=w651:bool[])
                    n215 = And Array Elements(Boolean array=w651) -> (logical AND=w649:bool)
                    n216 = case shown="真" w649 {
                      selector: w649 -> [_ w656]
                      tunnel: w648 -> [w655 w658]
                      tunnel: [w655 w657] -> w647
                      tunnel: [TRUE w656] -> w646
                      frame False {
                      }
                      frame True {
                        n217 = local write "完成"(w656) -> ()
                        n218 = local write "标定成功"(w656) -> ()
                        n219 = Increment(x=w658) -> (x+1=w657:i32)
                      }
                    }
                  }
                }
              }
            }
          }
        }
        frame "内部软件版本号" {
        }
        frame "客户软件版本号" {
        }
      }
    }
  }
